vi "process.vi"(8 "error in (no error)":errorcluster, 11 "img_name":string="path") -> (0 "error out":errorcluster, 2 "返回值":bool)   [LabVIEW 2019]
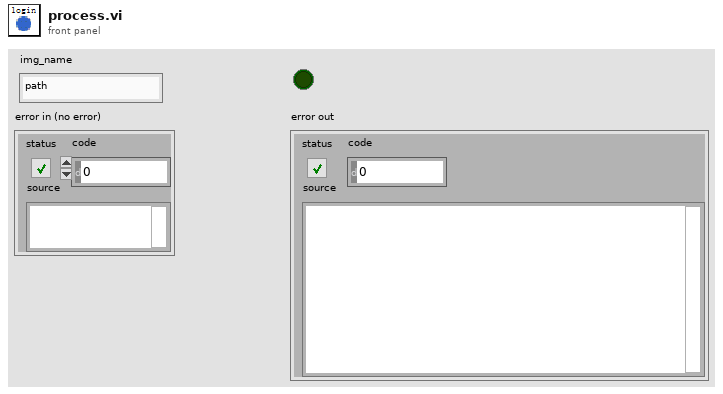
[diagram p1: front panel]
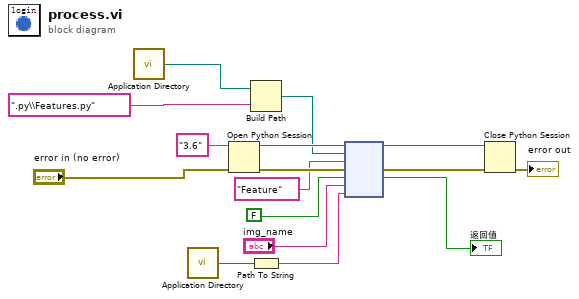
[diagram p0: block diagram]
diagram:
  n1 = call <vilib>:"Application Directory.vi"() -> ("Application Directory"=w3:path)
  n2 = call <vilib>:"Application Directory.vi"() -> ("Application Directory"=w6:path)
  n3 = Open Python Session(python version="3.6" ("Python version"), 3:"error in (no error)") -> (session out=w16:refnum<k35>, error out=w14:errorcluster)  [unwired: 1 in]
  n4 = Build Path(base path=w3, name or relative path=".py\\Features.py") -> (appended path=w1:path)
  n5 = Path To String(path=w6) -> (string=w5:string)
  n6 = node(w16, w1, "Feature" ("function name"), w14, FALSE, "img_name", w5) -> (w15:refnum<k35>, w13:errorcluster, →"返回值":bool)  [unwired: 2 in, 2 out]
  n7 = Close Python Session(session in=w15, error in=w13) -> (11:→"error out":errorcluster)
